vi "Facade.vi"(0 "Data In":T4, 2 "Display State In":T2, 3 "Container State":T3) -> (6 "Data Out":T4, 7 "Display State Out":T2, 8 "Action":T1)   [LabVIEW 2020, in "Slack.xctl"]
uses:
  Slack.xctl
  Data.vi
  Typedefs/Slack-Configuration.ctl
  Typedefs/Slack-User.ctl
  <vilib>/_xctls/Container State.ctl
  State.vi
  <vilib>/_xctls/Action.ctl
  <vilib>/_xctls/XControlSupport.lvlib
panel:
  out "Tab":enum32{"Page 1", "Page 2"}(tab)
  out "Name":string
  out "Workspace":string
  in  "Sign in Button":bool
types:
  T1 = typedef "XControlSupport.lvlib/Action.ctl" = cluster{"Data Changed?":bool, "State Changed?":bool, "Action Name":string}
  T2 = typedef "Slack.xctl/State.vi" = cluster{"client_id":string, "client_secret":string}
  T3 = typedef "XControlSupport.lvlib/Container State.ctl" = cluster{"Indicator?":bool, "Run Mode?":bool, " Refnum":refnum<vi>}
  T4 = typedef "Slack.xctl/Data.vi" = cluster{"config":T5, "users":T6[]}
  T5 = typedef "Slack-Configuration.ctl" = cluster{"app_id":string, "authed_user":cluster{"id":string}, "access_token":string, "bot_user_id":string, "team":cluster{"id":string, "name":string}, "bot channel":cluster{"id":string, "name":string}, "bot_user_name":string}
  T6 = typedef "Slack-User.ctl" = cluster{"id":string, "name":string}
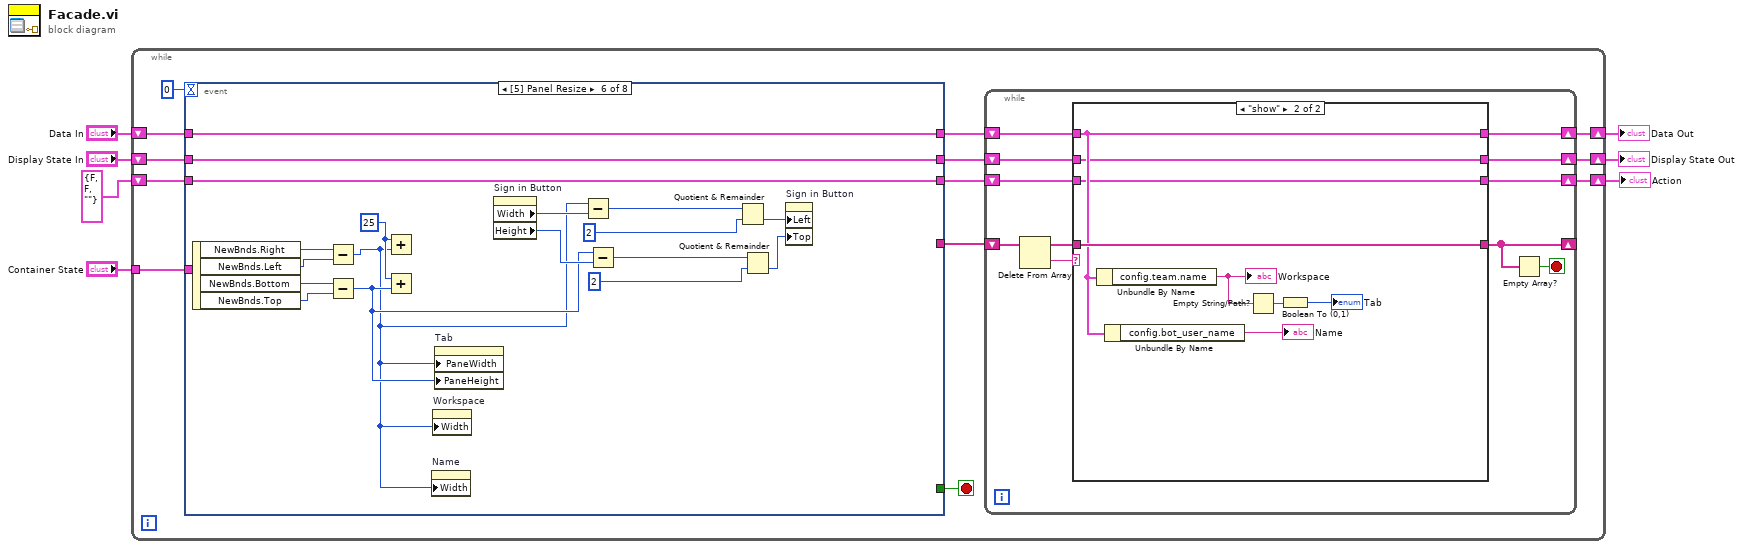
[diagram p0: block diagram]
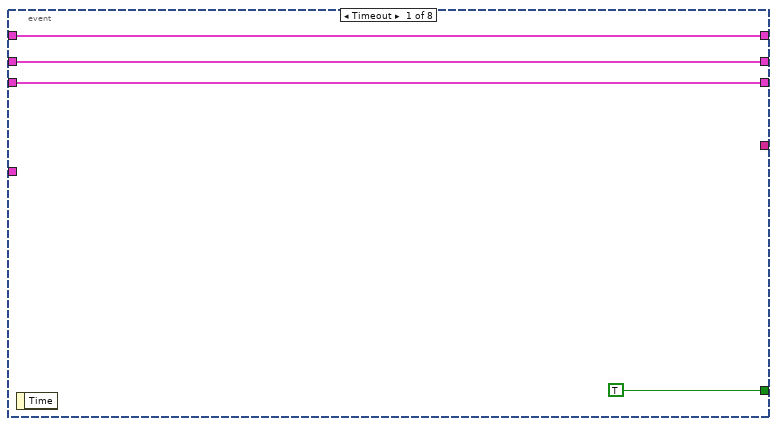
[diagram p2: hidden frame]
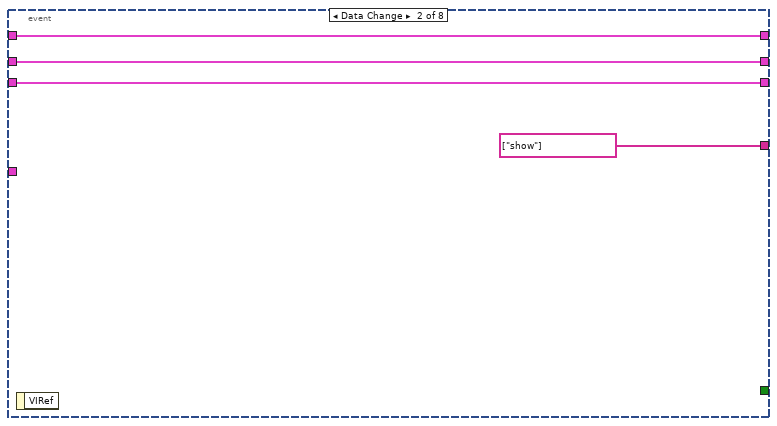
[diagram p3: hidden frame]
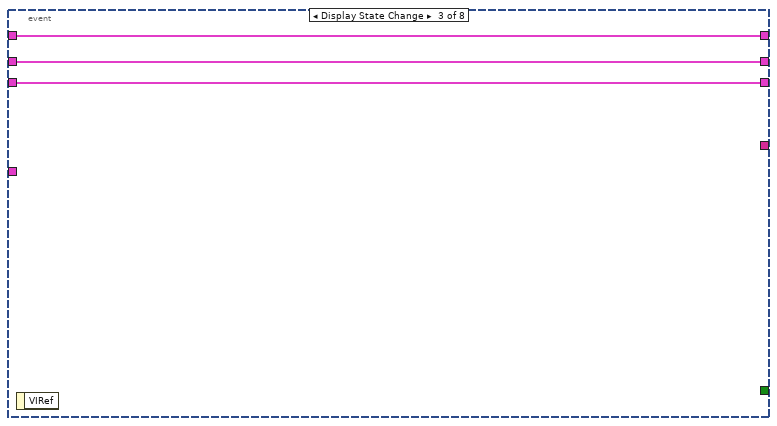
[diagram p4: hidden frame]
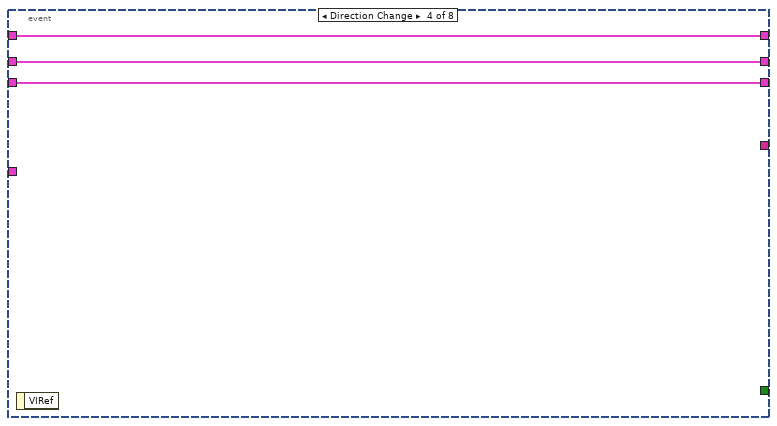
[diagram p5: hidden frame]
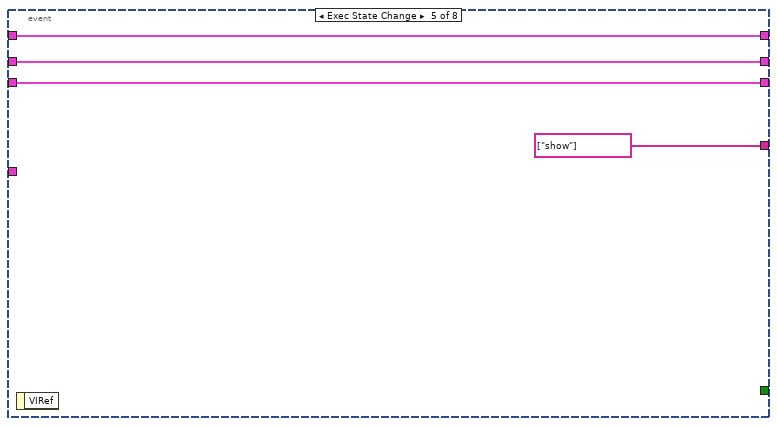
[diagram p6: hidden frame]
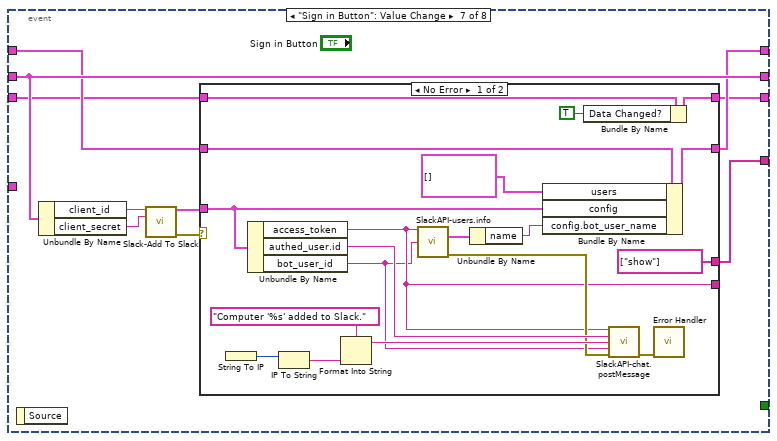
[diagram p7: hidden frame]
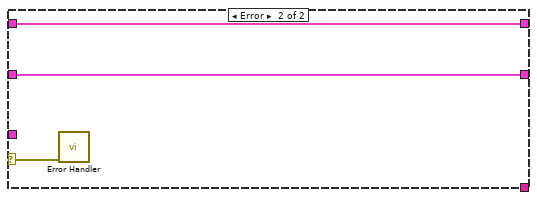
[diagram p8: hidden frame]
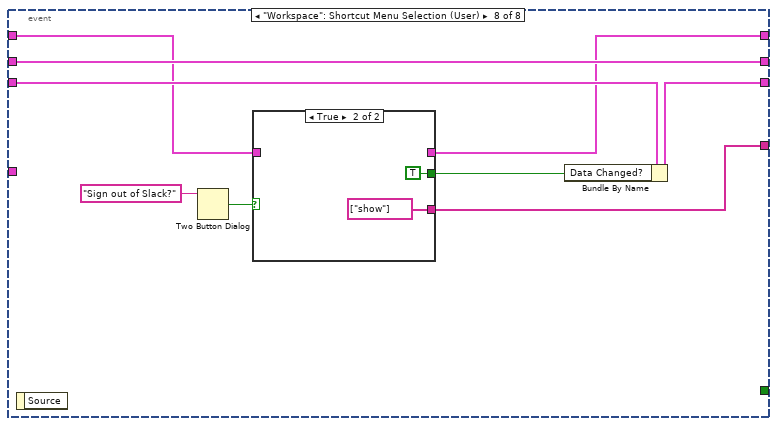
[diagram p9: hidden frame]
diagram:
  n1 = while {
    shift-right: [w9] -> w4
    shift-left: "Display State In" -> [w20]
    tunnel: "Container State" -> [w17]
    shift-right: [w10] -> w7
    shift-left: "Data In" -> [w16]
    shift-right: [w8] -> w2
    shift-left: T1 {"Data Changed?"=FALSE, "State Changed?"=FALSE, "Action Name"=""} ("Action") -> [w15]
    stop <- w19 stop-if-true
    n2 = event shown="[5] Panel Resize" {
      selector: _ -> [_ _ _ _ _ _ _ _]
      dyn-events: _ -> [_ _ _ _ _ _ _ _]
      timeout: 0 -> [_ _ _ _ _ _ _ _]
      tunnel: w20 -> [w22 w28 w31 w34 w38 w56 w66 w97]
      tunnel: [w22 w28 w31 w34 w38 w56 w66 w97] -> w12
      tunnel: [TRUE _ _ _ _ _ _ _] -> w19
      tunnel: w17 -> [_ _ _ _ _ _ _ _]
      tunnel: w16 -> [w21 w25 w30 w33 w37 w55 w62 w93]
      tunnel: [w21 w25 w30 w33 w37 w55 w61 w92] -> w13
      tunnel: [w23 w27 w29 w32 w36 w54 w57 w91] -> w11
      tunnel: w15 -> [w23 w27 w29 w32 w36 w54 w58 w96]
      tunnel: [_ string[] ["show"] _ _ string[] ["show"] _ w59 w89] -> w14
      event Timeout {
        n3 = event-data() -> ()  [unwired: 1 in, 1 out]
      }
      event Data Change {
        n4 = event-data() -> ()  [unwired: 1 in, 1 out]
      }
      event Display State Change {
        n5 = event-data() -> ()  [unwired: 1 in, 1 out]
      }
      event Direction Change {
        n6 = event-data() -> ()  [unwired: 1 in, 1 out]
      }
      event Exec State Change {
        n7 = event-data() -> ()  [unwired: 1 in, 1 out]
      }
      event Panel Resize {
        w50 = 25
        n8 = event-data() -> ("NewBnds.Right"=w53:i16, "NewBnds.Left"=w49:i16, "NewBnds.Bottom"=w52:i16, "NewBnds.Top"=w51:i16)  [unwired: 1 in]
        n9 = Subtract(x=w53, y=w49) -> (x-y=w39:i16)
        n10 = Subtract(x=w52, y=w51) -> (x-y=w41:i16)
        n11 = Add(x=w50, y=w39) -> ()  [unwired: 1 out]
        n12 = Add(x=w50, y=w41) -> ()  [unwired: 1 out]
        n13 = property on="Name" class="Str"("Width"=w39) -> ()  [unwired: 2 in, 2 out]
        n14 = property on="Workspace" class="Str"("Width"=w39) -> ()  [unwired: 2 in, 2 out]
        n15 = property on="Tab" class="TabCtl (strict)"("PaneWidth"=w39, "PaneHeight"=w41) -> ()  [unwired: 2 in, 2 out]
        n16 = property on="Sign in Button" class="Bool"() -> ("Width"=w48:u32, "Height"=w42:u32)  [unwired: 2 in, 2 out]
        n17 = Subtract(x=w39, y=w48) -> (x-y=w47:u32)
        n18 = Subtract(x=w41, y=w42) -> (x-y=w44:u32)
        n19 = Quotient & Remainder(x=w47, y=u32 2) -> (floor(x/y)=w45:u32)  [unwired: 1 out]
        n20 = Quotient & Remainder(x=w44, y=u32 2) -> (floor(x/y)=w40:u32)  [unwired: 1 out]
        n21 = property on="Sign in Button" class="Bool"("Left"=w45, "Top"=w40) -> ()  [unwired: 2 in, 2 out]
      }
      event "Sign in Button": Value Change {
        n22 = event-data() -> ()  [unwired: 1 in, 1 out]
        n23 = Unbundle By Name(w66) -> ("client_id"=w65:string, "client_secret"=w64:string)
        n24 = call "Slack-Add To Slack.vi"("client_id"=w65, "client_secret"=w64) -> ("config"=w60:T5, "error out"=w63:errorcluster)  [unwired: 12 in]
        n25 = case shown="No Error" w63 {
          selector: w63 -> [_ w87]
          tunnel: [w77 w88] -> w61
          tunnel: w62 -> [w80 w88]
          tunnel: w60 -> [w79 _]
          tunnel: [string[] ["show"] _] -> w59
          tunnel: w58 -> [w72 w86]
          tunnel: [w71 w86] -> w57
          tunnel: [w68 _] -> _
          frame No Error {
            n26 = String To IP() -> (0:w85:u32)  [unwired: 1 in]
            n27 = Unbundle By Name(w79) -> ("access_token"=w68:string, "authed_user.id"=w76:string, "bot_user_id"=w67:string)
            n28 = IP To String(2:w85) -> (0:w83:string)  [unwired: 1 in]
            n29 = Format Into String(format string="Computer '%s' added to Slack.", w83) -> (resulting string=w82:string)  [unwired: 2 in, 1 out]
            n30 = call "SlackAPI-users.info.vi"("token"=w68, "user"=w67) -> ("user"=w75:T6, "error out"=w69:errorcluster)  [unwired: 11 in, 1 out]
            n31 = Unbundle By Name(w75) -> ("name"=w74:string)
            n32 = Bundle By Name(cluster=w80, "users"=T6[] [], "config"=w79, "config.bot_user_name"=w74) -> (w77:T4)
            n33 = Bundle By Name(cluster=w72, "Data Changed?"=TRUE) -> (w71:T1)
            n34 = call "SlackAPI-chat.postMessage.vi"("access_token"=w68, "user ID"=w76, "message"=w82, "username"=w67, "error in (no error)"=w69) -> ("error out"=w81:errorcluster)  [unwired: 10 in]
            n35 = call "Error Handler.vi"("error in (no error)"=w81) -> ()  [unwired: 13 in, 2 out]
          }
          frame Error {
            n36 = call "Error Handler.vi"("error in (no error)"=w87) -> ()  [unwired: 13 in, 2 out]
          }
        }
      }
      event "Workspace": Shortcut Menu Selection (User) {
        n37 = event-data() -> ()  [unwired: 1 in, 1 out]
        n38 = Two Button Dialog(message="Sign out of Slack?" ("T button name (\"OK\")")) -> (T button?=w94:bool)  [unwired: 2 in]
        n39 = case shown="True" w94 {
          tunnel: w93 -> [w98 _]
          tunnel: [w98 _] -> w92
          tunnel: [_ TRUE] -> w90
          tunnel: [_ string[] ["show"]] -> w89
          frame False {
          }
          frame True {
          }
        }
        n40 = Bundle By Name(cluster=w96, "Data Changed?"=w90) -> (w91:T1)
      }
    }
    n41 = while {
      shift-right: [w108] -> _
      shift-left: w14 -> [w111]
      shift-right: [w102] -> w8
      shift-left: w11 -> [w104]
      shift-right: [w101] -> w9
      shift-left: w12 -> [w105]
      shift-right: [w103] -> w10
      shift-left: w13 -> [w106]
      stop <- w107 stop-if-true
      n42 = Delete From Array(array=w111) -> (deleted portion=w109:string, array with subset deleted=w110:string[])  [unwired: 2 in]
      n43 = case shown="\"show\"" w109 {
        tunnel: w110 -> [w115 w123]
        tunnel: [w115 w123] -> w108
        tunnel: w106 -> [w114 w121]
        tunnel: w105 -> [w112 w120]
        tunnel: w104 -> [w113 w119]
        tunnel: [w114 w121] -> w103
        tunnel: [w113 w119] -> w102
        tunnel: [w112 w120] -> w101
        frame "", Default {
        }
        frame "show" {
          n44 = Unbundle By Name(w121) -> ("config.team.name"=w118:string)
          "Workspace" <- w118
          n45 = Unbundle By Name(w121) -> ("config.bot_user_name"=→"Name":string)
          n46 = Empty String/Path?(string/path=w118) -> (empty?=w122:bool)
          n47 = Boolean To (0,1)(Boolean=w122) -> (0, 1=→"Tab":i16)
        }
      }
      n48 = Empty Array?(array=w108) -> (empty?=w107:bool)
    }
  }
  "Display State Out" <- w4
  "Data Out" <- w7
  "Action" <- w2
